vi "Shooter.vi"() -> ()   [LabVIEW 2016]
panel:
  in  "Shooter Speed Setpoint":dbl
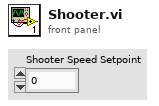
[diagram p1: front panel]
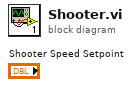
[diagram p0: block diagram]
diagram:
